vi "Init All Action Data.vi"(8 "Motor Labels":string[](array[string]), 9 "Action List":T2(array[cluster])=[{"Action Name"="Enable Motor", "JSON info"=[{"path"="Index", "data type"=enum."INT"}], "String Format"="%(Action Name) %(Index)"}, {"Action Name"="Disable Motor", "JSON info"=[{"path"="Index", "data type"=enum."INT"}], "String Format"="%(Action Name) %(Index)"}, {"Action Name"="Move Motor", "JSON info"=[{"path"="Index", "data type"=enum."INT"}, {"path"="Destination", "data type"=enum."DBL"}], "String Format"="%(Action Name) %(Index) to %(Destination)"}], 10 "Array of Action Data (JSON)":string[](array[string]), 11 "Action Names":string[](array[string])) -> (2 "Array of Data Types":T1(array[cluster]), 3 "Array of Data Names&Defaults":cluster{"Data Names&Defaults":string[][]}[](array[cluster]))   [LabVIEW 2016, in "Hardware.lvlib" / "Motions.lvlib" / "Motions.lvclass"]
uses:
  <userlib>/Common Components/Hardware/Abstract System/Motions/Motions/Motions.lvclass
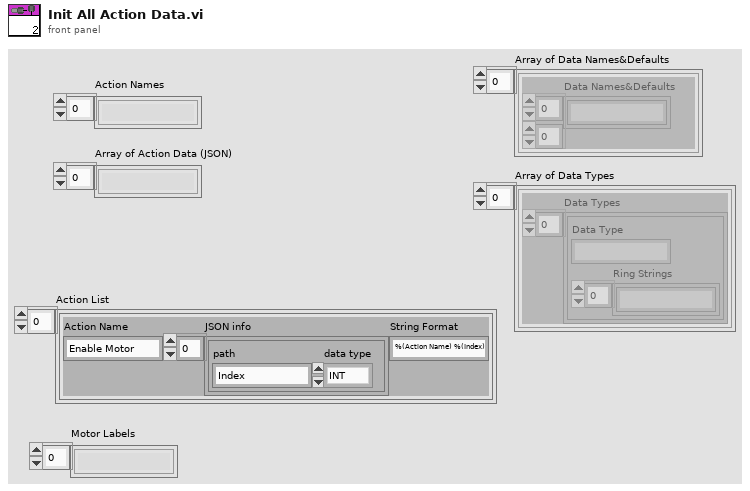
[diagram p1: front panel]
types:
  T1 = cluster{"Data Types":cluster{"Data Type":string, "Ring Strings":string[]}[]}[]
  T2 = cluster{"Action Name":string, "JSON info":cluster{"path":string, "data type":enum16{"INT", "DBL", "BOOL", "String"}}[], "String Format":string}[]
  T3 = cluster{"Data Type":string, "Ring Strings":string[]}[]
  T4 = cluster{"Data Types":cluster{"Data Type":string, "Ring Strings":string[]}[]}
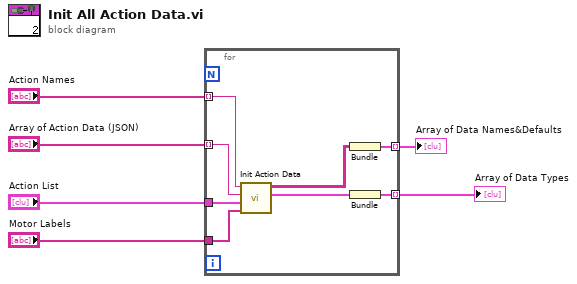
[diagram p0: block diagram]
diagram:
  n1 = for {
    tunnel: "Action Names" -> [w14] mode=indexing
    tunnel: "Array of Action Data (JSON)" -> [w13] mode=indexing
    tunnel: "Action List" -> [w12]
    tunnel: "Motor Labels" -> [w11]
    tunnel: [w9] -> w2 mode=indexing
    tunnel: [w7] -> w1 mode=indexing
    n2 = call <userlib>:"Init Action Data.vi"("Motor Labels"=w11, "Action List"=w12, "Action Data (JSON)"=w13, "Action Name"=w14) -> ("Data Types"=w8:T3, "Data Names&Defaults"=w10:string[][])  [unwired: 6 in]
    n3 = Bundle("Data Names&Defaults"=w10) -> (w9:cluster{"Data Names&Defaults":string[][]})  [unwired: 1 in]
    n4 = Bundle("Data Types"=w8) -> (w7:T4)  [unwired: 1 in]
  }
  "Array of Data Names&Defaults" <- w2
  "Array of Data Types" <- w1
